vi "GeoData.vi"() -> ()   [LabVIEW 2017] (continued)
County\tH1\n65257\t29089\tHigbee\tMO\tHoward County\tH1\n65230\t29089\tArmstrong\tMO\tHoward County\tH1\n65243\t29089\tClark\tMO\tHoward County\tH1\n65274\t29089\tNew franklin\tMO\tHoward County\tH1\n65793\t29091\tWillow springs\tMO\tHowell County\tH1\n65626\t29091\tCaulfield\tMO\tHowell County\tH1\n65637\t29091\tDora\tMO\tHowell County\tH1\n65688\t29091\tBrandsville\tMO\tHowell County\tH1\n65788\t29091\tPeace valley\tMO\tHowell County\tH1\n65689\t29091\tCabool\tMO\tHowell County\tH1\n65775\t29091\tWest plains\tMO\tHowell County\tH1\n65790\t29091\tPottersville\tMO\tHowell County\tH1\n65789\t29091\tPomona\tMO\tHowell County\tH1\n65609\t29091\tBakersfield\tMO\tHowell County\tH1\n65548\t29091\tMountain view\tMO\tHowell County\tH1\n65692\t29091\tKoshkonong\tMO\tHowell County\tH1\n65777\t29091\tMoody\tMO\tHowell County\tH1\n63624\t29093\tBismarck\tMO\tIron County\tH1\n63656\t29093\tMiddle brook\tMO\tIron County\tH1\n63620\t29093\tAnnapolis\tMO\tIron County\tH1\n63663\t29093\tPilot knob\tMO\tIron County\tH1\n63623\t29093\tBelleview\tMO\tIron County\tH1\n63636\t29093\tDes arc\tMO\tIron County\tH1\n63650\t29093\tIronton\tMO\tIron County\tH1\n63675\t29093\tVulcan\tMO\tIron County\tH1\n63621\t29093\tArcadia\tMO\tIron County\tH1\n65440\t29093\tBoss\tMO\tIron County\tH1\n63631\t29093\tCaledonia\tMO\tIron County\tH1\n65566\t29093\tViburnum\tMO\tIron County\tH1\n65439\t29093\tBixby\tMO\tIron County\tH1\n64137\t29095\tKansas city\tMO\tJackson County\tH1\n64111\t29095\tKansas city\tMO\tJackson County\tH1\n64053\t29095\tIndependence\tMO\tJackson County\tH1\n64055\t29095\tIndependence\tMO\tJackson County\tH1\n64064\t29095\tLees summit\tMO\tJackson County\tH1\n64029\t29095\tGrain valley\tMO\tJackson County\tH1\n64106\t29095\tKansas city\tMO\tJackson County\tH1\n64108\t29095\tKansas city\tMO\tJackson County\tH1\n64034\t29095\tGreenwood\tMO\tJackson County\tH1\n64118\t29095\tKansas city\tMO\tJackson County\tH1\n64136\t29095\tKansas city\tMO\tJackson County\tH1\n64139\t29095\tKansas city\tMO\tJackson County\tH1\n64125\t29095\tKansas city\tMO\tJackson County\tH1\n64030\t29095\tGrandview\tMO\tJackson County\tH1\n64014\t29095\tBlue springs\tMO\tJackson County\tH1\n64066\t29095\tLevasy\tMO\tJackson County\tH1\n64080\t29095\tPleasant hill\tMO\tJackson County\tH1\n64123\t29095\tKansas city\tMO\tJackson County\tH1\n64131\t29095\tKansas city\tMO\tJackson County\tH1\n64145\t29095\tKansas city\tMO\tJackson County\tH1\n64128\t29095\tKansas city\tMO\tJackson County\tH1\n64121\t29095\tKansas city\tMO\tJackson County\tH1\n64170\t29095\tKansas city\tMO\tJackson County\tH1\n64050\t29095\tIndependence\tMO\tJackson County\tH1\n64057\t29095\tIndependence\tMO\tJackson County\tH1\n64133\t29095\tKansas city\tMO\tJackson County\tH1\n64109\t29095\tKansas city\tMO\tJackson County\tH1\n64130\t29095\tKansas city\tMO\tJackson County\tH1\n64134\t29095\tKansas city\tMO\tJackson County\tH1\n64129\t29095\tKansas city\tMO\tJackson County\tH1\n64158\t29095\tKansas city\tMO\tJackson County\tH1\n64163\t29095\tKansas city\tMO\tJackson County\tH1\n64070\t29095\tLone jack\tMO\tJackson County\tH1\n64102\t29095\tKansas city\tMO\tJackson County\tH1\n64105\t29095\tKansas city\tMO\tJackson County\tH1\n64086\t29095\tLees summit\tMO\tJackson County\tH1\n64101\t29095\tKansas city\tMO\tJackson County\tH1\n64124\t29095\tKansas city\tMO\tJackson County\tH1\n64157\t29095\tKansas city\tMO\tJackson County\tH1\n64088\t29095\tSibley\tMO\tJackson County\tH1\n64061\t29095\tKingsville\tMO\tJackson County\tH1\n64051\t29095\tIndependence\tMO\tJackson County\tH1\n64002\t29095\tLees summit\tMO\tJackson County\tH1\n64081\t29095\tLees summit\tMO\tJackson County\tH1\n64013\t29095\tBlue springs\tMO\tJackson County\tH1\n64016\t29095\tBuckner\tMO\tJackson County\tH1\n64112\t29095\tKansas city\tMO\tJackson County\tH1\n64114\t29095\tKansas city\tMO\tJackson County\tH1\n64110\t29095\tKansas city\tMO\tJackson County\tH1\n64152\t29095\tKansas city\tMO\tJackson County\tH1\n64127\t29095\tKansas city\tMO\tJackson County\tH1\n64147\t29095\tKansas city\tMO\tJackson County\tH1\n64120\t29095\tKansas city\tMO\tJackson County\tH1\n64146\t29095\tKansas city\tMO\tJackson County\tH1\n64199\t29095\tKansas city\tMO\tJackson County\tH1\n64058\t29095\tIndependence\tMO\tJackson County\tH1\n64054\t29095\tIndependence\tMO\tJackson County\tH1\n64074\t29095\tNapoleon\tMO\tJackson County\tH1\n64119\t29095\tKansas city\tMO\tJackson County\tH1\n64138\t29095\tKansas city\tMO\tJackson County\tH1\n64149\t29095\tKansas city\tMO\tJackson County\tH1\n64156\t29095\tKansas city\tMO\tJackson County\tH1\n64132\t29095\tKansas city\tMO\tJackson County\tH1\n64171\t29095\tKansas city\tMO\tJackson County\tH1\n64148\t29095\tKansas city\tMO\tJackson County\tH1\n64141\t29095\tKansas city\tMO\tJackson County\tH1\n64999\t29095\tKansas city\tMO\tJackson County\tH1\n64052\t29095\tIndependence\tMO\tJackson County\tH1\n64015\t29095\tBlue springs\tMO\tJackson County\tH1\n64063\t29095\tLees summit\tMO\tJackson County\tH1\n64075\t29095\tOak grove\tMO\tJackson County\tH1\n64056\t29095\tIndependence\tMO\tJackson County\tH1\n64082\t29095\tLees summit\tMO\tJackson County\tH1\n64113\t29095\tKansas city\tMO\tJackson County\tH1\n64155\t29095\tKansas city\tMO\tJackson County\tH1\n64126\t29095\tKansas city\tMO\tJackson County\tH1\n64197\t29095\tKansas city\tMO\tJackson County\tH1\n64065\t29095\tLees summit\tMO\tJackson County\tH1\n64198\t29095\tKansas city\tMO\tJackson County\tH1\n64855\t29097\tOronogo\tMO\tJasper County\tH1\n64859\t29097\tReeds\tMO\tJasper County\tH1\n64873\t29097\tWentworth\tMO\tJasper County\tH1\n64804\t29097\tJoplin\tMO\tJasper County\tH1\n64832\t29097\tAsbury\tMO\tJasper County\tH1\n64848\t29097\tLa russell\tMO\tJasper County\tH1\n64849\t29097\tNeck city\tMO\tJasper County\tH1\n64834\t29097\tCarl junction\tMO\tJasper County\tH1\n64841\t29097\tDuenweg\tMO\tJasper County\tH1\n64862\t29097\tSarcoxie\tMO\tJasper County\tH1\n64835\t29097\tCarterville\tMO\tJasper County\tH1\n64840\t29097\tDiamond\tMO\tJasper County\tH1\n64801\t29097\tJoplin\tMO\tJasper County\tH1\n64748\t29097\tGolden city\tMO\tJasper County\tH1\n64857\t29097\tPurcell\tMO\tJasper County\tH1\n64833\t29097\tAvilla\tMO\tJasper County\tH1\n64802\t29097\tJoplin\tMO\tJasper County\tH1\n64803\t29097\tJoplin\tMO\tJasper County\tH1\n64830\t29097\tAlba\tMO\tJasper County\tH1\n64870\t29097\tWebb city\tMO\tJasper County\tH1\n64836\t29097\tCarthage\tMO\tJasper County\tH1\n64755\t29097\tJasper\tMO\tJasper County\tH1\n63051\t29099\tHouse springs\tMO\tJefferson County\tH1\n63050\t29099\tHillsboro\tMO\tJefferson County\tH1\n63070\t29099\tPevely\tMO\tJefferson County\tH1\n63061\t29099\tLuebbering\tMO\tJefferson County\tH1\n63057\t29099\tLiguori\tMO\tJefferson County\tH1\n63016\t29099\tCedar hill\tMO\tJefferson County\tH1\n63048\t29099\tHerculaneum\tMO\tJefferson County\tH1\n63627\t29099\tBloomsdale\tMO\tJefferson County\tH1\n63065\t29099\tMapaville\tMO\tJefferson County\tH1\n63628\t29099\tBonne terre\tMO\tJefferson County\tH1\n63012\t29099\tBarnhart\tMO\tJefferson County\tH1\n63026\t29099\tFenton\tMO\tJefferson County\tH1\n63049\t29099\tHigh ridge\tMO\tJefferson County\tH1\n63010\t29099\tArnold\tMO\tJefferson County\tH1\n63028\t29099\tFestus\tMO\tJefferson County\tH1\n63069\t29099\tPacific\tMO\tJefferson County\tH1\n63052\t29099\tImperial\tMO\tJefferson County\tH1\n63023\t29099\tDittmer\tMO\tJefferson County\tH1\n63020\t29099\tDe soto\tMO\tJefferson County\tH1\n63041\t29099\tGrubville\tMO\tJefferson County\tH1\n63015\t29099\tCatawissa\tMO\tJefferson County\tH1\n63019\t29099\tCrystal city\tMO\tJefferson County\tH1\n63030\t29099\tFletcher\tMO\tJefferson County\tH1\n63053\t29099\tKimmswick\tMO\tJefferson County\tH1\n63072\t29099\tRobertsville\tMO\tJefferson County\tH1\n63087\t29099\tValles mines\tMO\tJefferson County\tH1\n63025\t29099\tEureka\tMO\tJefferson County\tH1\n63066\t29099\tMorse mill\tMO\tJefferson County\tH1\n63047\t29099\tHematite\tMO\tJefferson County\tH1\n64076\t29101\tOdessa\tMO\tJohnson County\tH1\n64020\t29101\tConcordia\tMO\tJohnson County\tH1\n65351\t29101\tSweet springs\tMO\tJohnson County\tH1\n64011\t29101\tBates city\tMO\tJohnson County\tH1\n64071\t29101\tMayview\tMO\tJohnson County\tH1\n64093\t29101\tWarrensburg\tMO\tJohnson County\tH1\n64037\t29101\tHigginsville\tMO\tJohnson County\tH1\n64080\t29101\tPleasant hill\tMO\tJohnson County\tH1\n65336\t29101\tKnob noster\tMO\tJohnson County\tH1\n64070\t29101\tLone jack\tMO\tJohnson County\tH1\n64733\t29101\tChilhowee\tMO\tJohnson County\tH1\n65305\t29101\tWhiteman air force base\tMO\tJohnson County\tH1\n64061\t29101\tKingsville\tMO\tJohnson County\tH1\n65332\t29101\tGreen ridge\tMO\tJohnson County\tH1\n64019\t29101\tCenterview\tMO\tJohnson County\tH1\n64726\t29101\tBlairstown\tMO\tJohnson County\tH1\n64747\t29101\tGarden city\tMO\tJohnson County\tH1\n65337\t29101\tLa monte\tMO\tJohnson County\tH1\n65360\t29101\tWindsor\tMO\tJohnson County\tH1\n64761\t29101\tLeeton\tMO\tJohnson County\tH1\n64040\t29101\tHolden\tMO\tJohnson County\tH1\n63530\t29103\tAtlanta\tMO\tKnox County\tH1\n63460\t29103\tNovelty\tMO\tKnox County\tH1\n63458\t29103\tNewark\tMO\tKnox County\tH1\n63547\t29103\tHurdland\tMO\tKnox County\tH1\n63537\t29103\tEdina\tMO\tKnox County\tH1\n63531\t29103\tBaring\tMO\tKnox County\tH1\n63446\t29103\tKnox city\tMO\tKnox County\tH1\n65536\t29105\tLebanon\tMO\tLaclede County\tH1\n65470\t29105\tFalcon\tMO\tLaclede County\tH1\n65713\t29105\tNiangua\tMO\tLaclede County\tH1\n65632\t29105\tConway\tMO\tLaclede County\tH1\n65543\t29105\tLynchburg\tMO\tLaclede County\tH1\n65722\t29105\tPhillipsburg\tMO\tLaclede County\tH1\n65552\t29105\tPlato\tMO\tLaclede County\tH1\n65534\t29105\tLaquey\tMO\tLaclede County\tH1\n65567\t29105\tStoutland\tMO\tLaclede County\tH1\n65556\t29105\tRichland\tMO\tLaclede County\tH1\n65463\t29105\tEldridge\tMO\tLaclede County\tH1\n65662\t29105\tGrovespring\tMO\tLaclede County\tH1\n65590\t29105\tLong lane\tMO\tLaclede County\tH1\n65020\t29105\tCamdenton\tMO\tLaclede County\tH1\n64076\t29107\tOdessa\tMO\tLafayette County\tH1\n64020\t29107\tConcordia\tMO\tLafayette County\tH1\n65351\t29107\tSweet springs\tMO\tLafayette County\tH1\n64011\t29107\tBates city\tMO\tLafayette County\tH1\n64071\t29107\tMayview\tMO\tLafayette County\tH1\n64037\t29107\tHigginsville\tMO\tLafayette County\tH1\n64070\t29107\tLone jack\tMO\tLafayette County\tH1\n64067\t29107\tLexington\tMO\tLafayette County\tH1\n64022\t29107\tDover\tMO\tLafayette County\tH1\n64096\t29107\tWaverly\tMO\tLafayette County\tH1\n64074\t29107\tNapoleon\tMO\tLafayette County\tH1\n64017\t29107\tCamden\tMO\tLafayette County\tH1\n64075\t29107\tOak grove\tMO\tLafayette County\tH1\n64001\t29107\tAlma\tMO\tLafayette County\tH1\n64021\t29107\tCorder\tMO\tLafayette County\tH1\n64097\t29107\tWellington\tMO\tLafayette County\tH1\n65321\t29107\tBlackburn\tMO\tLafayette County\tH1\n64873\t29109\tWentworth\tMO\tLawrence County\tH1\n64848\t29109\tLa russell\tMO\tLawrence County\tH1\n65682\t29109\tLockwood\tMO\tLawrence County\tH1\n65705\t29109\tMarionville\tMO\tLawrence County\tH1\n65752\t29109\tSouth greenfield\tMO\tLawrence County\tH1\n65654\t29109\tFreistatt\tMO\tLawrence County\tH1\n64862\t29109\tSarcoxie\tMO\tLawrence County\tH1\n65610\t29109\tBillings\tMO\tLawrence County\tH1\n65604\t29109\tAsh grove\tMO\tLawrence County\tH1\n65738\t29109\tRepublic\tMO\tLawrence County\tH1\n65756\t29109\tStotts city\tMO\tLawrence County\tH1\n65664\t29109\tHalltown\tMO\tLawrence County\tH1\n65605\t29109\tAurora\tMO\tLawrence County\tH1\n65723\t29109\tPierce city\tMO\tLawrence County\tH1\n65646\t29109\tEverton\tMO\tLawrence County\tH1\n65612\t29109\tBois d arc\tMO\tLawrence County\tH1\n65708\t29109\tMonett\tMO\tLawrence County\tH1\n65769\t29109\tVerona\tMO\tLawrence County\tH1\n64748\t29109\tGolden city\tMO\tLawrence County\tH1\n65707\t29109\tMiller\tMO\tLawrence County\tH1\n65712\t29109\tMount vernon\tMO\tLawrence County\tH1\n63447\t29111\tLa belle\tMO\tLewis County\tH1\n63457\t29111\tMonticello\tMO\tLewis County\tH1\n63473\t29111\tWilliamstown\tMO\tLewis County\tH1\n63435\t29111\tCanton\tMO\tLewis County\tH1\n63452\t29111\tLewistown\tMO\tLewis County\tH1\n63448\t29111\tLa grange\tMO\tLewis County\tH1\n63438\t29111\tDurham\tMO\tLewis County\tH1\n63454\t29111\tMaywood\tMO\tLewis County\tH1\n63440\t29111\tEwing\tMO\tLewis County\tH1\n63446\t29111\tKnox city\tMO\tLewis County\tH1\n63471\t29111\tTaylor\tMO\tLewis County\tH1\n63381\t29113\tTruxton\tMO\tLincoln County\tH1\n63369\t29113\tOld monroe\tMO\tLincoln County\tH1\n63347\t29113\tFoley\tMO\tLincoln County\tH1\n63390\t29113\tWright city\tMO\tLincoln County\tH1\n63348\t29113\tForistell\tMO\tLincoln County\tH1\n63333\t29113\tBellflower\tMO\tLincoln County\tH1\n63377\t29113\tSilex\tMO\tLincoln County\tH1\n63379\t29113\tTroy\tMO\tLincoln County\tH1\n63389\t29113\tWinfield\tMO\tLincoln County\tH1\n63344\t29113\tEolia\tMO\tLincoln County\tH1\n63362\t29113\tMoscow mills\tMO\tLincoln County\tH1\n63383\t29113\tWarrenton\tMO\tLincoln County\tH1\n63349\t29113\tHawk point\tMO\tLincoln County\tH1\n63359\t29113\tMiddletown\tMO\tLincoln County\tH1\n63334\t29113\tBowling green\tMO\tLincoln County\tH1\n63343\t29113\tElsberry\tMO\tLincoln County\tH1\n63387\t29113\tWhiteside\tMO\tLincoln County\tH1\n64653\t29115\tLinneus\tMO\tLinn County\tH1\n65281\t29115\tSalisbury\tMO\tLinn County\tH1\n64658\t29115\tMarceline\tMO\tLinn County\tH1\n64688\t29115\tWheeling\tMO\tLinn County\tH1\n64651\t29115\tLaclede\tMO\tLinn County\tH1\n64674\t29115\tPurdin\tMO\tLinn County\tH1\n63566\t29115\tWinigan\tMO\tLinn County\tH1\n64631\t29115\tBucklin\tMO\tLinn County\tH1\n64628\t29115\tBrookfield\tMO\tLinn County\tH1\n64635\t29115\tChula\tMO\tLinn County\tH1\n63557\t29115\tNew boston\tMO\tLinn County\tH1\n65261\t29115\tKeytesville\tMO\tLinn County\tH1\n64652\t29115\tLaredo\tMO\tLinn County\tH1\n64646\t29115\tHumphreys\tMO\tLinn County\tH1\n64659\t29115\tMeadville\tMO\tLinn County\tH1\n64630\t29115\tBrowning\tMO\tLinn County\tH1\n64681\t29115\tSumner\tMO\tLinn County\tH1\n64643\t29117\tHale\tMO\tLivingston County\tH1\n64664\t29117\tMooresville\tMO\tLivingston County\tH1\n64656\t29117\tLudlow\tMO\tLivingston County\tH1\n64688\t29117\tWheeling\tMO\tLivingston County\tH1\n64625\t29117\tBreckenridge\tMO\tLivingston County\tH1\n64601\t29117\tChillicothe\tMO\tLivingston County\tH1\n64648\t29117\tJamesport\tMO\tLivingston County\tH1\n64635\t29117\tChula\tMO\tLivingston County\tH1\n64638\t29117\tDawn\tMO\tLivingston County\tH1\n64624\t29117\tBraymer\tMO\tLivingston County\tH1\n64686\t29117\tUtica\tMO\tLivingston County\tH1\n64683\t29117\tTrenton\tMO\tLivingston County\tH1\n64850\t29119\tNeosho\tMO\tMcDonald County\tH1\n64847\t29119\tLanagan\tMO\tMcDonald County\tH1\n64868\t29119\tTiff city\tMO\tMcDonald County\tH1\n64863\t29119\tSouth west city\tMO\tMcDonald County\tH1\n65647\t29119\tExeter\tMO\tMcDonald County\tH1\n65730\t29119\tPowell\tMO\tMcDonald County\tH1\n64865\t29119\tSeneca\tMO\tMcDonald County\tH1\n64831\t29119\tAnderson\tMO\tMcDonald County\tH1\n64856\t29119\tPineville\tMO\tMcDonald County\tH1\n64861\t29119\tRocky comfort\tMO\tMcDonald County\tH1\n64843\t29119\tGoodman\tMO\tMcDonald County\tH1\n64867\t29119\tStella\tMO\tMcDonald County\tH1\n65772\t29119\tWashburn\tMO\tMcDonald County\tH1\n64854\t29119\tNoel\tMO\tMcDonald County\tH1\n65745\t29119\tSeligman\tMO\tMcDonald County\tH1\n63552\t29121\tMacon\tMO\tMacon County\tH1\n63530\t29121\tAtlanta\tMO\tMacon County\tH1\n65260\t29121\tJacksonville\tMO\tMacon County\tH1\n63539\t29121\tEthel\tMO\tMacon County\tH1\n63538\t29121\tElmer\tMO\tMacon County\tH1\n63532\t29121\tBevier\tMO\tMacon County\tH1\n65247\t29121\tExcello\tMO\tMacon County\tH1\n64658\t29121\tMarceline\tMO\tMacon County\tH1\n63431\t29121\tAnabel\tMO\tMacon County\tH1\n63534\t29121\tCallao\tMO\tMacon County\tH1\n64631\t29121\tBucklin\tMO\tMacon County\tH1\n63557\t29121\tNew boston\tMO\tMacon County\tH1\n63549\t29121\tLa plata\tMO\tMacon County\tH1\n63451\t29121\tLeonard\tMO\tMacon County\tH1\n63558\t29121\tNew cambria\tMO\tMacon County\tH1\n63437\t29121\tClarence\tMO\tMacon County\tH1\n63620\t29123\tAnnapolis\tMO\tMadison County\tH1\n63655\t29123\tMarquand\tMO\tMadison County\tH1\n63636\t29123\tDes arc\tMO\tMadison County\tH1\n63645\t29123\tFredericktown\tMO\tMadison County\tH1\n63650\t29123\tIronton\tMO\tMadison County\tH1\n63640\t29123\tFarmington\tMO\tMadison County\tH1\n63621\t29123\tArcadia\tMO\tMadison County\tH1\n65559\t29125\tSaint james\tMO\tMaries County\tH1\n65582\t29125\tVienna\tMO\tMaries County\tH1\n65580\t29125\tVichy\tMO\tMaries County\tH1\n65058\t29125\tMeta\tMO\tMaries County\tH1\n65401\t29125\tRolla\tMO\tMaries County\tH1\n65443\t29125\tBrinktown\tMO\tMaries County\tH1\n65013\t29125\tBelle\tMO\tMaries County\tH1\n65014\t29125\tBland\tMO\tMaries County\tH1\n65001\t29125\tArgyle\tMO\tMaries County\tH1\n65459\t29125\tDixon\tMO\tMaries County\tH1\n63456\t29127\tMonroe city\tMO\tMarion County\tH1\n63401\t29127\tHannibal\tMO\tMarion County\tH1\n63461\t29127\tPalmyra\tMO\tMarion County\tH1\n63443\t29127\tHunnewell\tMO\tMarion County\tH1\n63438\t29127\tDurham\tMO\tMarion County\tH1\n63463\t29127\tPhiladelphia\tMO\tMarion County\tH1\n63454\t29127\tMaywood\tMO\tMarion County\tH1\n63440\t29127\tEwing\tMO\tMarion County\tH1\n63439\t29127\tEmden\tMO\tMarion County\tH1\n63471\t29127\tTaylor\tMO\tMarion County\tH1\n64673\t29129\tPrinceton\tMO\tMercer County\tH1\n64679\t29129\tSpickard\tMO\tMercer County\tH1\n64632\t29129\tCainsville\tMO\tMercer County\tH1\n64672\t29129\tPowersville\tMO\tMercer County\tH1\n64661\t29129\tMercer\tMO\tMercer County\tH1\n64667\t29129\tNewtown\tMO\tMercer County\tH1\n64645\t29129\tHarris\tMO\tMercer County\tH1\n65452\t29131\tCrocker\tMO\tMiller County\tH1\n65065\t29131\tOsage beach\tMO\tMiller County\tH1\n65082\t29131\tTuscumbia\tMO\tMiller County\tH1\n65032\t29131\tEugene\tMO\tMiller County\tH1\n65047\t29131\tKaiser\tMO\tMiller County\tH1\n65072\t29131\tRocky mount\tMO\tMiller County\tH1\n65017\t29131\tBrumley\tMO\tMiller County\tH1\n65058\t29131\tMeta\tMO\tMiller County\tH1\n65079\t29131\tSunrise beach\tMO\tMiller County\tH1\n65591\t29131\tMontreal\tMO\tMiller County\tH1\n65040\t29131\tHenley\tMO\tMiller County\tH1\n65486\t29131\tIberia\tMO\tMiller County\tH1\n65083\t29131\tUlman\tMO\tMiller County\tH1\n65026\t29131\tEldon\tMO\tMiller County\tH1\n65074\t29131\tRussellville\tMO\tMiller County\tH1\n65459\t29131\tDixon\tMO\tMiller County\tH1\n65075\t29131\tSaint elizabeth\tMO\tMiller County\tH1\n65049\t29131\tLake ozark\tMO\tMiller County\tH1\n65064\t29131\tOlean\tMO\tMiller County\tH1\n63845\t29133\tEast prairie\tMO\tMississippi County\tH1\n63882\t29133\tWyatt\tMO\tMississippi County\tH1\n63881\t29133\tWolf island\tMO\tMississippi County\tH1\n63834\t29133\tCharleston\tMO\tMississippi County\tH1\n63801\t29133\tSikeston\tMO\tMississippi County\tH1\n63823\t29133\tBertrand\tMO\tMississippi County\tH1\n63820\t29133\tAnniston\tMO\tMississippi County\tH1\n65011\t29135\tBarnett\tMO\tMoniteau County\tH1\n65287\t29135\tWooldridge\tMO\tMoniteau County\tH1\n65081\t29135\tTipton\tMO\tMoniteau County\tH1\n65084\t29135\tVersailles\tMO\tMoniteau County\tH1\n65055\t29135\tMc girk\tMO\tMoniteau County\tH1\n65034\t29135\tFortuna\tMO\tMoniteau County\tH1\n65018\t29135\tCalifornia\tMO\tMoniteau County\tH1\n65023\t29135\tCentertown\tMO\tMoniteau County\tH1\n65050\t29135\tLatham\tMO\tMoniteau County\tH1\n65025\t29135\tClarksburg\tMO\tMoniteau County\tH1\n65026\t29135\tEldon\tMO\tMoniteau County\tH1\n65074\t29135\tRussellville\tMO\tMoniteau County\tH1\n65068\t29135\tPrairie home\tMO\tMoniteau County\tH1\n65042\t29135\tHigh point\tMO\tMoniteau County\tH1\n65046\t29135\tJamestown\tMO\tMoniteau County\tH1\n65064\t29135\tOlean\tMO\tMoniteau County\tH1\n65260\t29137\tJacksonville\tMO\tMonroe County\tH1\n63456\t29137\tMonroe city\tMO\tMonroe County\tH1\n65263\t29137\tMadison\tMO\tMonroe County\tH1\n65265\t29137\tMexico\tMO\tMonroe County\tH1\n65282\t29137\tSanta fe\tMO\tMonroe County\tH1\n63468\t29137\tShelbina\tMO\tMonroe County\tH1\n65240\t29137\tCentralia\tMO\tMonroe County\tH1\n65258\t29137\tHolliday\tMO\tMonroe County\tH1\n63443\t29137\tHunnewell\tMO\tMonroe County\tH1\n65270\t29137\tMoberly\tMO\tMonroe County\tH1\n63437\t29137\tClarence\tMO\tMonroe County\tH1\n63462\t29137\tPerry\tMO\tMonroe County\tH1\n65275\t29137\tParis\tMO\tMonroe County\tH1\n65243\t29137\tClark\tMO\tMonroe County\tH1\n65283\t29137\tStoutsville\tMO\tMonroe County\tH1\n63381\t29139\tTruxton\tMO\tMontgomery County\tH1\n65069\t29139\tRhineland\tMO\tMontgomery County\tH1\n63351\t29139\tJonesburg\tMO\tMontgomery County\tH1\n63363\t29139\tNew florence\tMO\tMontgomery County\tH1\n63350\t29139\tHigh hill\tMO\tMontgomery County\tH1\n63333\t29139\tBellflower\tMO\tMontgomery County\tH1\n63384\t29139\tWellsville\tMO\tMontgomery County\tH1\n65041\t29139\tHermann\tMO\tMontgomery County\tH1\n63359\t29139\tMiddletown\tMO\tMontgomery County\tH1\n63361\t29139\tMontgomery city\tMO\tMontgomery County\tH1\n65264\t29139\tMartinsburg\tMO\tMontgomery County\tH1\n65011\t29141\tBarnett\tMO\tMorgan County\tH1\n65329\t29141\tFlorence\tMO\tMorgan County\tH1\n65081\t29141\tTipton\tMO\tMorgan County\tH1\n65084\t29141\tVersailles\tMO\tMorgan County\tH1\n65350\t29141\tSmithton\tMO\tMorgan County\tH1\n65037\t29141\tGravois mills\tMO\tMorgan County\tH1\n65034\t29141\tFortuna\tMO\tMorgan County\tH1\n65072\t29141\tRocky mount\tMO\tMorgan County\tH1\n65038\t29141\tLaurie\tMO\tMorgan County\tH1\n65079\t29141\tSunrise beach\tMO\tMorgan County\tH1\n65325\t29141\tCole camp\tMO\tMorgan County\tH1\n65078\t29141\tStover\tMO\tMorgan County\tH1\n65026\t29141\tEldon\tMO\tMorgan County\tH1\n65074\t29141\tRussellville\tMO\tMorgan County\tH1\n65348\t29141\tOtterville\tMO\tMorgan County\tH1\n65345\t29141\tMora\tMO\tMorgan County\tH1\n65354\t29141\tSyracuse\tMO\tMorgan County\tH1\n63867\t29143\tMatthews\tMO\tNew Madrid County\tH1\n63874\t29143\tRisco\tMO\tNew Madrid County\tH1\n63845\t29143\tEast prairie\tMO\tNew Madrid County\tH1\n63822\t29143\tBernie\tMO\tNew Madrid County\tH1\n63833\t29143\tCatron\tMO\tNew Madrid County\tH1\n63878\t29143\tTallapoosa\tMO\tNew Madrid County\tH1\n63866\t29143\tMarston\tMO\tNew Madrid County\tH1\n63801\t29143\tSikeston\tMO\tNew Madrid County\tH1\n63828\t29143\tCanalou\tMO\tNew Madrid County\tH1\n63860\t29143\tKewanee\tMO\tNew Madrid County\tH1\n63870\t29143\tParma\tMO\tNew Madrid County\tH1\n63873\t29143\tPortageville\tMO\tNew Madrid County\tH1\n63837\t29143\tClarkton\tMO\tNew Madrid County\tH1\n63862\t29143\tLilbourn\tMO\tNew Madrid County\tH1\n63868\t29143\tMorehouse\tMO\tNew Madrid County\tH1\n63869\t29143\tNew madrid\tMO\tNew Madrid County\tH1\n63848\t29143\tGideon\tMO\tNew Madrid County\tH1\n64850\t29145\tNeosho\tMO\tNewton County\tH1\n64873\t29145\tWentworth\tMO\tNewton County\tH1\n64804\t29145\tJoplin\tMO\tNewton County\tH1\n64865\t29145\tSeneca\tMO\tNewton County\tH1\n64862\t29145\tSarcoxie\tMO\tNewton County\tH1\n64861\t29145\tRocky comfort\tMO\tNewton County\tH1\n64844\t29145\tGranby\tMO\tNewton County\tH1\n64843\t29145\tGoodman\tMO\tNewton County\tH1\n64840\t29145\tDiamond\tMO\tNewton County\tH1\n65723\t29145\tPierce city\tMO\tNewton County\tH1\n64801\t29145\tJoplin\tMO\tNewton County\tH1\n64864\t29145\tSaginaw\tMO\tNewton County\tH1\n64867\t29145\tStella\tMO\tNewton County\tH1\n64866\t29145\tStark city\tMO\tNewton County\tH1\n64858\t29145\tRacine\tMO\tNewton County\tH1\n64842\t29145\tFairview\tMO\tNewton County\tH1\n65734\t29145\tPurdy\tMO\tNewton County\tH1\n64461\t29147\tHopkins\tMO\tNodaway County\tH1\n64455\t29147\tGraham\tMO\tNodaway County\tH1\n64486\t29147\tSheridan\tMO\tNodaway County\tH1\n64434\t29147\tConception junction\tMO\tNodaway County\tH1\n64468\t29147\tMaryville\tMO\tNodaway County\tH1\n64431\t29147\tClearmont\tMO\tNodaway County\tH1\n64475\t29147\tParnell\tMO\tNodaway County\tH1\n64489\t29147\tStanberry\tMO\tNodaway County\tH1\n64432\t29147\tClyde\tMO\tNodaway County\tH1\n64445\t29147\tElmo\tMO\tNodaway County\tH1\n64433\t29147\tConception\tMO\tNodaway County\tH1\n64428\t29147\tBurlington junction\tMO\tNodaway County\tH1\n64423\t29147\tBarnard\tMO\tNodaway County\tH1\n64427\t29147\tBolckow\tMO\tNodaway County\tH1\n64476\t29147\tPickering\tMO\tNodaway County\tH1\n64479\t29147\tRavenwood\tMO\tNodaway County\tH1\n64457\t29147\tGuilford\tMO\tNodaway County\tH1\n64487\t29147\tSkidmore\tMO\tNodaway County\tH1\n65606\t29149\tAlton\tMO\tOregon County\tH1\n65778\t29149\tMyrtle\tMO\tOregon County\tH1\n65791\t29149\tThayer\tMO\tOregon County\tH1\n65692\t29149\tKoshkonong\tMO\tOregon County\tH1\n65690\t29149\tCouch\tMO\tOregon County\tH1\n65035\t29151\tFreeburg\tMO\tOsage County\tH1\n65062\t29151\tMount sterling\tMO\tOsage County\tH1\n65051\t29151\tLinn\tMO\tOsage County\tH1\n65582\t29151\tVienna\tMO\tOsage County\tH1\n65058\t29151\tMeta\tMO\tOsage County\tH1\n65101\t29151\tJefferson city\tMO\tOsage County\tH1\n65076\t29151\tSaint thomas\tMO\tOsage County\tH1\n65016\t29151\tBonnots mill\tMO\tOsage County\tH1\n65013\t29151\tBelle\tMO\tOsage County\tH1\n65014\t29151\tBland\tMO\tOsage County\tH1\n65001\t29151\tArgyle\tMO\tOsage County\tH1\n65048\t29151\tKoeltztown\tMO\tOsage County\tH1\n65061\t29151\tMorrison\tMO\tOsage County\tH1\n65054\t29151\tLoose creek\tMO\tOsage County\tH1\n65024\t29151\tChamois\tMO\tOsage County\tH1\n65085\t29151\tWestphalia\tMO\tOsage County\tH1\n65626\t29153\tCaulfield\tMO\tOzark County\tH1\n65761\t29153\tTheodosia\tMO\tOzark County\tH1\n65729\t29153\tPontiac\tMO\tOzark County\tH1\n65784\t29153\tZanoni\tMO\tOzark County\tH1\n65637\t29153\tDora\tMO\tOzark County\tH1\n65676\t29153\tIsabella\tMO\tOzark County\tH1\n65741\t29153\tRockbridge\tMO\tOzark County\tH1\n65638\t29153\tDrury\tMO\tOzark County\tH1\n65766\t29153\tUdall\tMO\tOzark County\tH1\n65618\t29153\tBrixey\tMO\tOzark County\tH1\n65790\t29153\tPottersville\tMO\tOzark County\tH1\n65773\t29153\tWasola\tMO\tOzark County\tH1\n65608\t29153\tAva\tMO\tOzark County\tH1\n65666\t29153\tHardenville\tMO\tOzark County\tH1\n65733\t29153\tProtem\tMO\tOzark County\tH1\n65762\t29153\tThornfield\tMO\tOzark County\tH1\n65755\t29153\tSquires\tMO\tOzark County\tH1\n65655\t29153\tGainesville\tMO\tOzark County\tH1\n65760\t29153\tTecumseh\tMO\tOzark County\tH1\n65609\t29153\tBakersfield\tMO\tOzark County\tH1\n65715\t29153\tNoble\tMO\tOzark County\tH1\n63857\t29155\tKennett\tMO\tPemiscot County\tH1\n63830\t29155\tCaruthersville\tMO\tPemiscot County\tH1\n63879\t29155\tWardell\tMO\tPemiscot County\tH1\n63840\t29155\tDeering\tMO\tPemiscot County\tH1\n63877\t29155\tSteele\tMO\tPemiscot County\tH1\n63851\t29155\tHayti\tMO\tPemiscot County\tH1\n63873\t29155\tPortageville\tMO\tPemiscot County\tH1\n63855\t29155\tHornersville\tMO\tPemiscot County\tH1\n63827\t29155\tBragg city\tMO\tPemiscot County\tH1\n63839\t29155\tCooter\tMO\tPemiscot County\tH1\n63849\t29155\tGobler\tMO\tPemiscot County\tH1\n63853\t29155\tHolland\tMO\tPemiscot County\tH1\n63852\t29155\tHolcomb\tMO\tPemiscot County\tH1\n63826\t29155\tBraggadocio\tMO\tPemiscot County\tH1\n63746\t29157\tFarrar\tMO\tPerry County\tH1\n63732\t29157\tAltenburg\tMO\tPerry County\tH1\n63737\t29157\tBrazeau\tMO\tPerry County\tH1\n63783\t29157\tUniontown\tMO\tPerry County\tH1\n63645\t29157\tFredericktown\tMO\tPerry County\tH1\n63748\t29157\tFrohna\tMO\tPerry County\tH1\n63673\t29157\tSaint mary\tMO\tPerry County\tH1\n63770\t29157\tOld appleton\tMO\tPerry County\tH1\n63775\t29157\tPerryville\tMO\tPerry County\tH1\n63781\t29157\tSedgewickville\tMO\tPerry County\tH1\n63776\t29157\tMc bride\tMO\tPerry County\tH1\n65340\t29159\tMarshall\tMO\tPettis County\tH1\n64020\t29159\tConcordia\tMO\tPettis County\tH1\n65350\t29159\tSmithton\tMO\tPettis County\tH1\n65351\t29159\tSweet springs\tMO\tPettis County\tH1\n65336\t29159\tKnob noster\tMO\tPettis County\tH1\n65347\t29159\tNelson\tMO\tPettis County\tH1\n65301\t29159\tSedalia\tMO\tPettis County\tH1\n65325\t29159\tCole camp\tMO\tPettis County\tH1\n65333\t29159\tHoustonia\tMO\tPettis County\tH1\n65078\t29159\tStover\tMO\tPettis County\tH1\n65332\t29159\tGreen ridge\tMO\tPettis County\tH1\n65302\t29159\tSedalia\tMO\tPettis County\tH1\n65337\t29159\tLa monte\tMO\tPettis County\tH1\n65360\t29159\tWindsor\tMO\tPettis County\tH1\n65334\t29159\tHughesville\tMO\tPettis County\tH1\n65348\t29159\tOtterville\tMO\tPettis County\tH1\n65345\t29159\tMora\tMO\tPettis County\tH1\n65335\t29159\tIonia\tMO\tPettis County\tH1\n65559\t29161\tSaint james\tMO\tPhelps County\tH1\n65550\t29161\tNewburg\tMO\tPhelps County\tH1\n65461\t29161\tDuke\tMO\tPhelps County\tH1\n65409\t29161\tRolla\tMO\tPhelps County\tH1\n65401\t29161\tRolla\tMO\tPhelps County\tH1\n65402\t29161\tRolla\tMO\tPhelps County\tH1\n65462\t29161\tEdgar springs\tMO\tPhelps County\tH1\n65436\t29161\tBeulah\tMO\tPhelps County\tH1\n65560\t29161\tSalem\tMO\tPhelps County\tH1\n65453\t29161\tCuba\tMO\tPhelps County\tH1\n65542\t29161\tLicking\tMO\tPhelps County\tH1\n65459\t29161\tDixon\tMO\tPhelps County\tH1\n65529\t29161\tJerome\tMO\tPhelps County\tH1\n65449\t29161\tCook sta\tMO\tPhelps County\tH1\n63339\t29163\tCurryville\tMO\tPike County\tH1\n63441\t29163\tFrankford\tMO\tPike County\tH1\n63336\t29163\tClarksville\tMO\tPike County\tH1\n63344\t29163\tEolia\tMO\tPike County\tH1\n63459\t29163\tNew london\tMO\tPike County\tH1\n63382\t29163\tVandalia\tMO\tPike County\tH1\n63353\t29163\tLouisiana\tMO\tPike County\tH1\n63359\t29163\tMiddletown\tMO\tPike County\tH1\n63334\t29163\tBowling green\tMO\tPike County\tH1\n63343\t29163\tElsberry\tMO\tPike County\tH1\n63433\t29163\tAshburn\tMO\tPike County\tH1\n63330\t29163\tAnnada\tMO\tPike County\tH1\n64439\t29165\tDearborn\tMO\tPlatte County\tH1\n64118\t29165\tKansas city\tMO\tPlatte County\tH1\n64150\t29165\tRiverside\tMO\tPlatte County\tH1\n64154\t29165\tKansas city\tMO\tPlatte County\tH1\n64151\t29165\tKansas city\tMO\tPlatte County\tH1\n64089\t29165\tSmithville\tMO\tPlatte County\tH1\n64133\t29165\tKansas city\tMO\tPlatte County\tH1\n64163\t29165\tKansas city\tMO\tPlatte County\tH1\n64444\t29165\tEdgerton\tMO\tPlatte County\tH1\n64018\t29165\tCamden point\tMO\tPlatte County\tH1\n64164\t29165\tKansas city\tMO\tPlatte County\tH1\n64079\t29165\tPlatte city\tMO\tPlatte County\tH1\n64028\t29165\tFarley\tMO\tPlatte County\tH1\n64440\t29165\tDe kalb\tMO\tPlatte County\tH1\n64153\t29165\tKansas city\tMO\tPlatte County\tH1\n64152\t29165\tKansas city\tMO\tPlatte County\tH1\n64484\t29165\tRushville\tMO\tPlatte County\tH1\n64190\t29165\tKansas city\tMO\tPlatte County\tH1\n64098\t29165\tWeston\tMO\tPlatte County\tH1\n64155\t29165\tKansas city\tMO\tPlatte County\tH1\n64492\t29165\tTrimble\tMO\tPlatte County\tH1\n64168\t29165\tKansas city\tMO\tPlatte County\tH1\n64092\t29165\tWaldron\tMO\tPlatte County\tH1\n65622\t29167\tBuffalo\tMO\tPolk County\tH1\n65645\t29167\tMorrisville\tMO\tPolk County\tH1\n65601\t29167\tAldrich\tMO\tPolk County\tH1\n65650\t29167\tFlemington\tMO\tPolk County\tH1\n65674\t29167\tHumansville\tMO\tPolk County\tH1\n65725\t29167\tPleasant hope\tMO\tPolk County\tH1\n65770\t29167\tWalnut grove\tMO\tPolk County\tH1\n65649\t29167\tFair play\tMO\tPolk County\tH1\n65663\t29167\tHalf way\tMO\tPolk County\tH1\n65724\t29167\tPittsburg\tMO\tPolk County\tH1\n65781\t29167\tWillard\tMO\tPolk County\tH1\n65648\t29167\tFair grove\tMO\tPolk County\tH1\n65727\t29167\tPolk\tMO\tPolk County\tH1\n65640\t29167\tDunnegan\tMO\tPolk County\tH1\n65613\t29167\tBolivar\tMO\tPolk County\tH1\n65767\t29167\tUrbana\tMO\tPolk County\tH1\n65710\t29167\tMorrisville\tMO\tPolk County\tH1\n65617\t29167\tBrighton\tMO\tPolk County\tH1\n65685\t29167\tLouisburg\tMO\tPolk County\tH1\n65473\t29169\tFort leonard wood\tMO\tPulaski County\tH1\n65452\t29169\tCrocker\tMO\tPulaski County\tH1\n65584\t29169\tSaint robert\tMO\tPulaski County\tH1\n65550\t29169\tNewburg\tMO\tPulaski County\tH1\n65461\t29169\tDuke\tMO\tPulaski County\tH1\n65552\t29169\tPlato\tMO\tPulaski County\tH1\n65457\t29169\tDevils elbow\tMO\tPulaski County\tH1\n65534\t29169\tLaquey\tMO\tPulaski County\tH1\n65556\t29169\tRichland\tMO\tPulaski County\tH1\n65583\t29169\tWaynesville\tMO\tPulaski County\tH1\n65459\t29169\tDixon\tMO\tPulaski County\tH1\n63560\t29171\tPollock\tMO\tPutnam County\tH1\n63559\t29171\tNovinger\tMO\tPutnam County\tH1\n63565\t29171\tUnionville\tMO\tPutnam County\tH1\n64672\t29171\tPowersville\tMO\tPutnam County\tH1\n64667\t29171\tNewtown\tMO\tPutnam County\tH1\n64655\t29171\tLucerne\tMO\tPutnam County\tH1\n63567\t29171\tWorthington\tMO\tPutnam County\tH1\n63551\t29171\tLivonia\tMO\tPutnam County\tH1\n63561\t29171\tQueen city\tMO\tPutnam County\tH1\n63544\t29171\tGreen castle\tMO\tPutnam County\tH1\n63456\t29173\tMonroe city\tMO\tRalls County\tH1\n63401\t29173\tHannibal\tMO\tRalls County\tH1\n63441\t29173\tFrankford\tMO\tRalls County\tH1\n63461\t29173\tPalmyra\tMO\tRalls County\tH1\n63459\t29173\tNew london\tMO\tRalls County\tH1\n63436\t29173\tCenter\tMO\tRalls County\tH1\n63382\t29173\tVandalia\tMO\tRalls County\tH1\n63352\t29173\tLaddonia\tMO\tRalls County\tH1\n63467\t29173\tSaverton\tMO\tRalls County\tH1\n63462\t29173\tPerry\tMO\tRalls County\tH1\n65260\t29175\tJacksonville\tMO\tRandolph County\tH1\n65263\t29175\tMadison\tMO\tRandolph County\tH1\n65259\t29175\tHuntsville\tMO\tRandolph County\tH1\n65244\t29175\tClifton hill\tMO\tRandolph County\tH1\n65247\t29175\tExcello\tMO\tRandolph County\tH1\n65281\t29175\tSalisbury\tMO\tRandolph County\tH1\n63534\t29175\tCallao\tMO\tRandolph County\tH1\n65270\t29175\tMoberly\tMO\tRandolph County\tH1\n65278\t29175\tRenick\tMO\tRandolph County\tH1\n65257\t29175\tHigbee\tMO\tRandolph County\tH1\n65239\t29175\tCairo\tMO\tRandolph County\tH1\n65230\t29175\tArmstrong\tMO\tRandolph County\tH1\n65243\t29175\tClark\tMO\tRandolph County\tH1\n64671\t29177\tPolo\tMO\tRay County\tH1\n64085\t29177\tRichmond\tMO\tRay County\tH1\n64024\t29177\tExcelsior springs\tMO\tRay County\tH1\n64077\t29177\tOrrick\tMO\tRay County\tH1\n64035\t29177\tHardin\tMO\tRay County\tH1\n64637\t29177\tCowgill\tMO\tRay County\tH1\n64062\t29177\tLawson\tMO\tRay County\tH1\n64624\t29177\tBraymer\tMO\tRay County\tH1\n64668\t29177\tNorborne\tMO\tRay County\tH1\n64017\t29177\tCamden\tMO\tRay County\tH1\n64084\t29177\tRayville\tMO\tRay County\tH1\n64036\t29177\tHenrietta\tMO\tRay County\tH1\n63638\t29179\tEllington\tMO\tReynolds County\tH1\n63665\t29179\tRedford\tMO\tReynolds County\tH1\n63629\t29179\tBunker\tMO\tReynolds County\tH1\n63965\t29179\tVan buren\tMO\tReynolds County\tH1\n63620\t29179\tAnnapolis\tMO\tReynolds County\tH1\n63957\t29179\tPiedmont\tMO\tReynolds County\tH1\n63650\t29179\tIronton\tMO\tReynolds County\tH1\n63633\t29179\tCenterville\tMO\tReynolds County\tH1\n63654\t29179\tLesterville\tMO\tReynolds County\tH1\n63625\t29179\tBlack\tMO\tReynolds County\tH1\n63666\t29179\tReynolds\tMO\tReynolds County\tH1\n63955\t29181\tOxly\tMO\tRipley County\tH1\n63942\t29181\tGatewood\tMO\tRipley County\tH1\n63931\t29181\tBriar\tMO\tRipley County\tH1\n63935\t29181\tDoniphan\tMO\tRipley County\tH1\n63953\t29181\tNaylor\tMO\tRipley County\tH1\n63939\t29181\tFairdealing\tMO\tRipley County\tH1\n63385\t29183\tWentzville\tMO\tSt. Charles County\tH1\n63366\t29183\tO fallon\tMO\tSt. Charles County\tH1\n63338\t29183\tCottleville\tMO\tSt. Charles County\tH1\n63301\t29183\tSaint charles\tMO\tSt. Charles County\tH1\n63376\t29183\tSaint peters\tMO\tSt. Charles County\tH1\n63373\t29183\tPortage des sioux\tMO\tSt. Charles County\tH1\n63348\t29183\tForistell\tMO\tSt. Charles County\tH1\n63302\t29183\tSaint charles\tMO\tSt. Charles County\tH1\n63346\t29183\tFlinthill\tMO\tSt. Charles County\tH1\n63303\t29183\tSaint charles\tMO\tSt. Charles County\tH1\n63365\t29183\tNew melle\tMO\tSt. Charles County\tH1\n63332\t29183\tAugusta\tMO\tSt. Charles County\tH1\n63367\t29183\tLake saint louis\tMO\tSt. Charles County\tH1\n63386\t29183\tWest alton\tMO\tSt. Charles County\tH1\n63304\t29183\tSaint charles\tMO\tSt. Charles County\tH1\n63368\t29183\tO fallon\tMO\tSt. Charles County\tH1\n63357\t29183\tMarthasville\tMO\tSt. Charles County\tH1\n63341\t29183\tDefiance\tMO\tSt. Charles County\tH1\n64780\t29185\tRockville\tMO\tSt. Clair County\tH1\n65785\t29185\tStockton\tMO\tSt. Clair County\tH1\n64740\t29185\tDeepwater\tMO\tSt. Clair County\tH1\n64763\t29185\tLowry city\tMO\tSt. Clair County\tH1\n65674\t29185\tHumansville\tMO\tSt. Clair County\tH1\n64783\t29185\tSchell city\tMO\tSt. Clair County\tH1\n64738\t29185\tCollins\tMO\tSt. Clair County\tH1\n64724\t29185\tAppleton city\tMO\tSt. Clair County\tH1\n64776\t29185\tOsceola\tMO\tSt. Clair County\tH1\n64744\t29185\tEl dorado springs\tMO\tSt. Clair County\tH1\n64781\t29185\tRoscoe\tMO\tSt. Clair County\tH1\n65774\t29185\tWeaubleau\tMO\tSt. Clair County\tH1\n64770\t29185\tMontrose\tMO\tSt. Clair County\tH1\n63627\t29186\tBloomsdale\tMO\tSte. Genevieve County\tH1\n63645\t29186\tFredericktown\tMO\tSte. Genevieve County\tH1\n63628\t29186\tBonne terre\tMO\tSte. Genevieve County\tH1\n63640\t29186\tFarmington\tMO\tSte. Genevieve County\tH1\n63673\t29186\tSaint mary\tMO\tSte. Genevieve County\tH1\n63028\t29186\tFestus\tMO\tSte. Genevieve County\tH1\n63036\t29186\tFrench village\tMO\tSte. Genevieve County\tH1\n63670\t29186\tSainte genevieve\tMO\tSte. Genevieve County\tH1\n63624\t29187\tBismarck\tMO\tSt. Francois County\tH1\n63653\t29187\tLeadwood\tMO\tSt. Francois County\tH1\n63648\t29187\tIrondale\tMO\tSt. Francois County\tH1\n63645\t29187\tFredericktown\tMO\tSt. Francois County\tH1\n63601\t29187\tPark hills\tMO\tSt. Francois County\tH1\n63650\t29187\tIronton\tMO\tSt. Francois County\tH1\n63628\t29187\tBonne terre\tMO\tSt. Francois County\tH1\n63651\t29187\tKnob lick\tMO\tSt. Francois County\tH1\n63640\t29187\tFarmington\tMO\tSt. Francois County\tH1\n63630\t29187\tCadet\tMO\tSt. Francois County\tH1\n63028\t29187\tFestus\tMO\tSt. Francois County\tH1\n63654\t29187\tLesterville\tMO\tSt. Francois County\tH1\n63036\t29187\tFrench village\tMO\tSt. Francois County\tH1\n63020\t29187\tDe soto\tMO\tSt. Francois County\tH1\n63626\t29187\tBlackwell\tMO\tSt. Francois County\tH1\n63637\t29187\tDoe run\tMO\tSt. Francois County\tH1\n63087\t29187\tValles mines\tMO\tSt. Francois County\tH1\n63074\t29189\tSaint ann\tMO\tSt. Louis County\tH1\n63105\t29189\tSaint louis\tMO\tSt. Louis County\tH1\n63034\t29189\tFlorissant\tMO\tSt. Louis County\tH1\n63044\t29189\tBridgeton\tMO\tSt. Louis County\tH1\n63043\t29189\tMaryland heights\tMO\tSt. Louis County\tH1\n63119\t29189\tSaint louis\tMO\tSt. Louis County\tH1\n63122\t29189\tSaint louis\tMO\tSt. Louis County\tH1\n63088\t29189\tValley park\tMO\tSt. Louis County\tH1\n63131\t29189\tSaint louis\tMO\tSt. Louis County\tH1\n63144\t29189\tSaint louis\tMO\tSt. Louis County\tH1\n63032\t29189\tFlorissant\tMO\tSt. Louis County\tH1\n63145\t29189\tSaint louis\tMO\tSt. Louis County\tH1\n63123\t29189\tSaint louis\tMO\tSt. Louis County\tH1\n63136\t29189\tSaint louis\tMO\tSt. Louis County\tH1\n63137\t29189\tSaint louis\tMO\tSt. Louis County\tH1\n63124\t29189\tSaint louis\tMO\tSt. Louis County\tH1\n63038\t29189\tWildwood\tMO\tSt. Louis County\tH1\n63040\t29189\tWildwood\tMO\tSt. Louis County\tH1\n63114\t29189\tSaint louis\tMO\tSt. Louis County\tH1\n63132\t29189\tSaint louis\tMO\tSt. Louis County\tH1\n63146\t29189\tSaint louis\tMO\tSt. Louis County\tH1\n63129\t29189\tSaint louis\tMO\tSt. Louis County\tH1\n63134\t29189\tSaint louis\tMO\tSt. Louis County\tH1\n63151\t29189\tSaint louis\tMO\tSt. Louis County\tH1\n63005\t29189\tChesterfield\tMO\tSt. Louis County\tH1\n63017\t29189\tChesterfield\tMO\tSt. Louis County\tH1\n63024\t29189\tBallwin\tMO\tSt. Louis County\tH1\n63031\t29189\tFlorissant\tMO\tSt. Louis County\tH1\n63120\t29189\tSaint louis\tMO\tSt. Louis County\tH1\n63143\t29189\tSaint louis\tMO\tSt. Louis County\tH1\n63125\t29189\tSaint louis\tMO\tSt. Louis County\tH1\n63128\t29189\tSaint louis\tMO\tSt. Louis County\tH1\n63026\t29189\tFenton\tMO\tSt. Louis County\tH1\n63049\t29189\tHigh ridge\tMO\tSt. Louis County\tH1\n63127\t29189\tSaint louis\tMO\tSt. Louis County\tH1\n63135\t29189\tSaint louis\tMO\tSt. Louis County\tH1\n63171\t29189\tSaint louis\tMO\tSt. Louis County\tH1\n63033\t29189\tFlorissant\tMO\tSt. Louis County\tH1\n63069\t29189\tPacific\tMO\tSt. Louis County\tH1\n
